vi "Analog Output Control Panel (No Objects).vi"(8 "error in (no error)":errorcluster) -> (0 "error out":errorcluster)   [LabVIEW 2009]
doc: "(Dynamic) A user-level application that simulates the physical front panel of the Instrument. Provide the user with buttons to manually control features of the instrument, and provide indicators of its current state."
uses:
  <vilib>/DAQmx/create/channels.llb/DAQmx Create Channel (AO-Voltage-Basic).vi
  <vilib>/DAQmx/write.llb/DAQmx Write (Analog DBL 1Chan 1Samp).vi
  Program Files/National Instruments/LabVIEW 2009/resource/objmgr/daqmx.rc
panel:
  in  "Copy actual to set":bool
  in  "Populate fields with member data":bool
  out "Ch1 voltage":dbl[unit]
  out "Ch1 lower limit":dbl[unit]
  out "Ch1 upper limit":dbl[unit]
  out "Ch0 voltage":dbl[unit]
  out "Ch0 lower limit":dbl[unit]
  out "Ch0 upper limit":dbl[unit]
  in  "Set Ch1 Voltage":bool
  in  "Set Ch0 Voltage":bool
  in  "Ch1 voltage set":dbl[unit]
  in  "Ch1 lower limit set":dbl[unit] min=-10.0 max=10.0
  in  "Ch1 upper limit set":dbl[unit] min=-10.0 max=10.0
  in  "Ch0 voltage set":dbl[unit]
  in  "Ch0 lower limit set":dbl[unit] min=-10.0 max=10.0
  in  "Ch0 upper limit set":dbl[unit] min=-10.0 max=10.0
  in  "Set Parameters":bool
  in  "Read to Control":bool
  in  "Read Parameters":bool
  in  "stop":bool
  # "We cannot read in the currently set voltage values !"
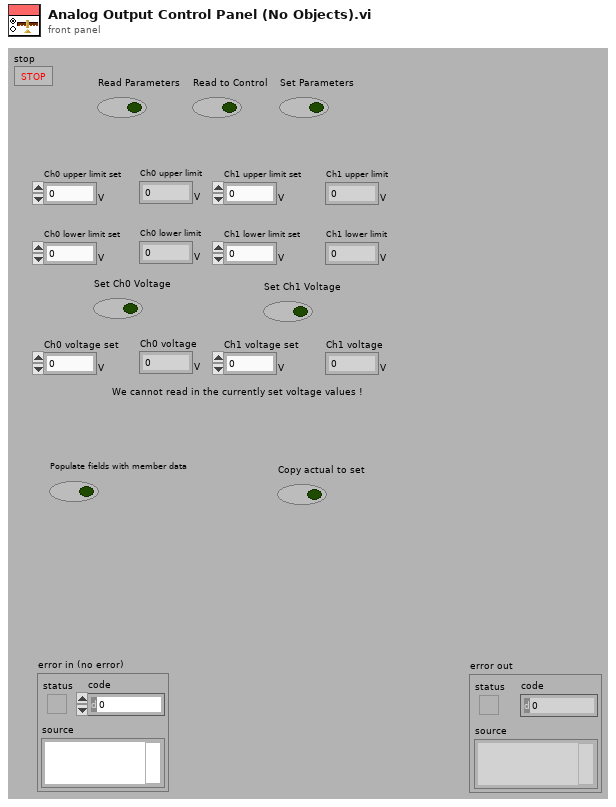
[diagram p1: front panel]
types:
  T1 = cluster{"Ch0":cluster{"Voltage":dbl[unit], "Max value":dbl[unit], "Min value":dbl[unit], "Ch 0 task":refnum<k21>}, "Ch1":cluster{"Voltage":dbl[unit], "Max value":dbl[unit], "Min value":dbl[unit], "Ch 1 task":refnum<k21>}}
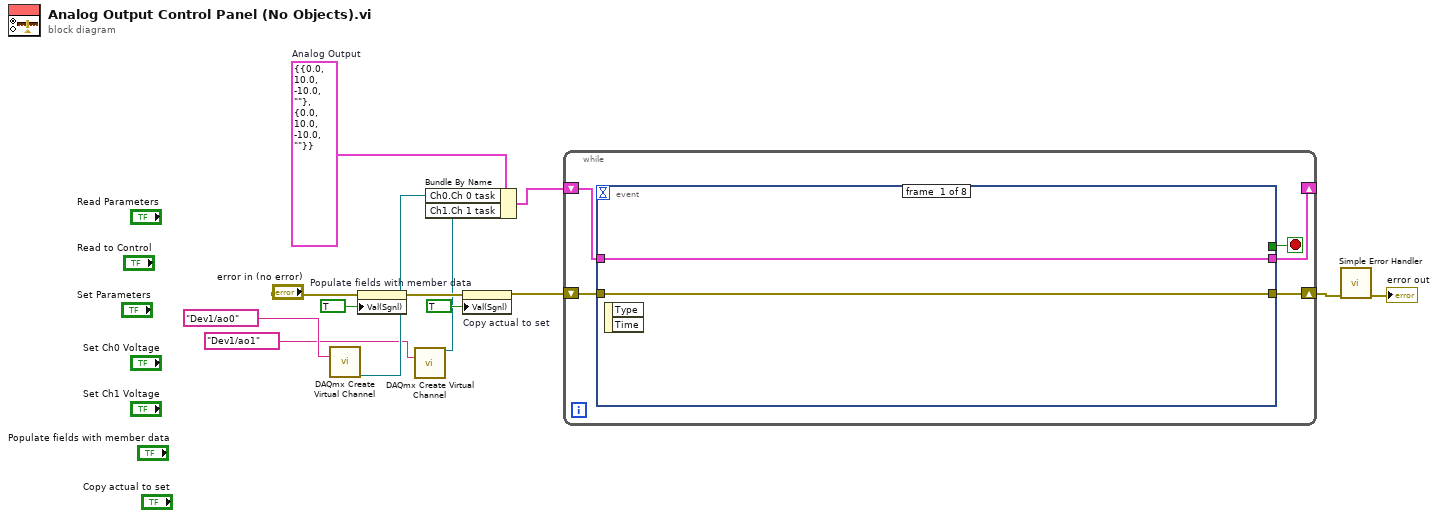
[diagram p0: block diagram]
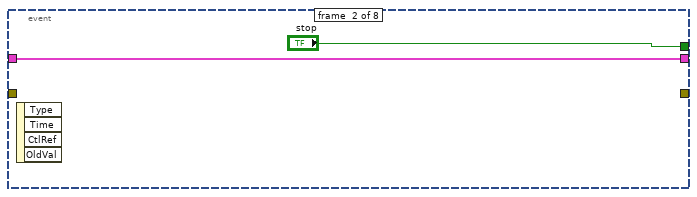
[diagram p2: hidden frame]
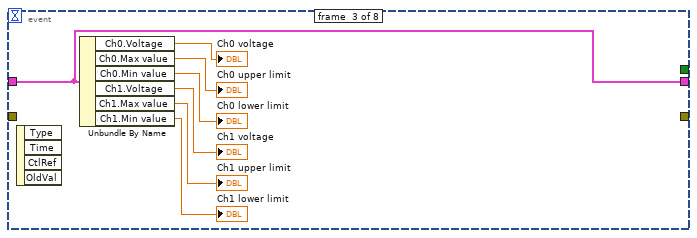
[diagram p3: hidden frame]
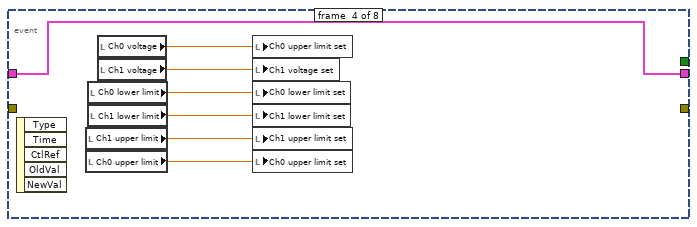
[diagram p4: hidden frame]
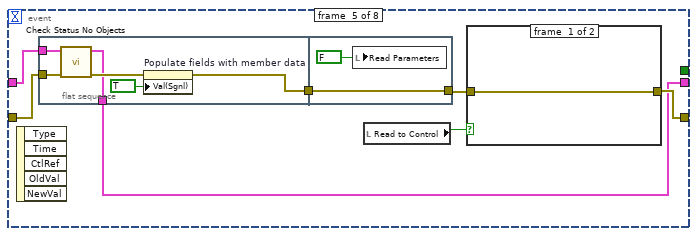
[diagram p5: hidden frame]
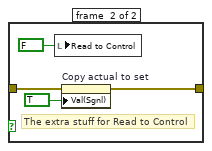
[diagram p6: hidden frame]
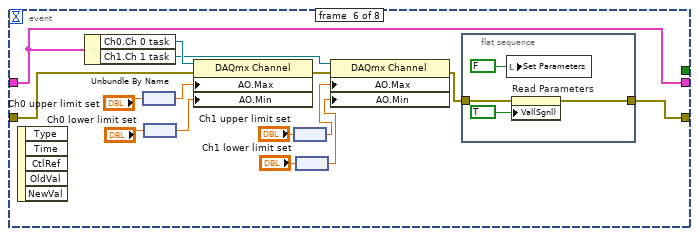
[diagram p7: hidden frame]
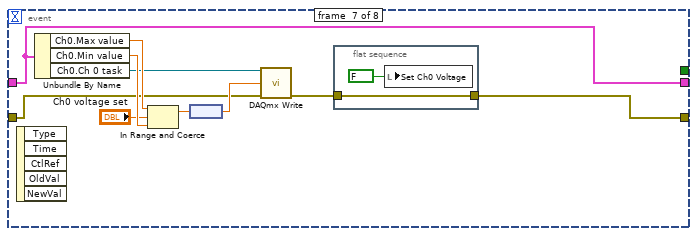
[diagram p8: hidden frame]
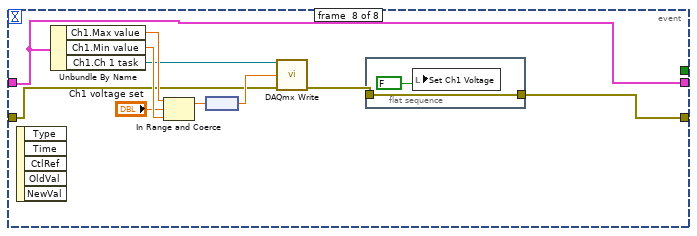
[diagram p9: hidden frame]
diagram:
  w6 = T1 {"Ch0"={"Voltage"=0.0, "Max value"=10.0, "Min value"=-10.0, "Ch 0 task"=""}, "Ch1"={"Voltage"=0.0, "Max value"=10.0, "Min value"=-10.0, "Ch 1 task"=""}}  # Analog Output
  n1 = call-poly <vilib>:"DAQmx Create Virtual Channel.vi"("physical channels"=tag "Dev1/ao0") -> ("task out"=w4:refnum<k21>)  [unwired: 13 in, 1 out]
  n2 = property on="Populate fields with member data" class="Bool (strict)"(error in="error in (no error)", "Val(Sgnl)"=TRUE ("Value (Signaling)")) -> (error out=w11:errorcluster)  [unwired: 1 in, 1 out]
  n3 = call-poly <vilib>:"DAQmx Create Virtual Channel.vi"("physical channels"=tag "Dev1/ao1") -> ("task out"=w3:refnum<k21>)  [unwired: 13 in, 1 out]
  n4 = Bundle By Name(cluster=w6, "Ch0.Ch 0 task"=w4, "Ch1.Ch 1 task"=w3) -> (w5:T1)
  n5 = property on="Copy actual to set" class="Bool (strict)"(error in=w11, "Val(Sgnl)"=TRUE ("Value (Signaling)")) -> (error out=w10:errorcluster)  [unwired: 1 in, 1 out]
  n6 = while {
    shift-right: [w14] -> _
    shift-left: w5 -> [w17]
    shift-right: [w16] -> w9
    shift-left: w10 -> [w18]
    stop <- w15 stop-if-true
    n7 = event shown="[4] \"Read Parameters\", \"Read to Control\": Value Change" {
      selector: _ -> [_ _ _ _ _ _ _ _]
      dyn-events: _ -> [_ _ _ _ _ _ _ _]
      timeout: _ -> [_ _ _ _ _ _ _ _]
      tunnel: [w20 _ _ _ w38 w57 w76 w88] -> w16
      tunnel: w18 -> [w20 _ _ _ w42 w71 w80 w92]
      tunnel: w17 -> [w19 w22 w23 w30 w43 w58 w77 w89]
      tunnel: [w19 w22 w23 w30 w37 w58 w77 w89] -> w14
      tunnel: [_ "stop" _ _ _ _ _ _] -> w15
      event #0 {
        n8 = event-data() -> ()  [unwired: 1 in, 2 out]
      }
      event #1 {
        n9 = event-data() -> ()  [unwired: 1 in, 4 out]
      }
      event #2 {
        n10 = event-data() -> ()  [unwired: 1 in, 4 out]
        n11 = Unbundle By Name(w23) -> ("Ch0.Voltage"=→"Ch0 voltage":dbl[unit], "Ch0.Max value"=→"Ch0 upper limit":dbl[unit], "Ch0.Min value"=→"Ch0 lower limit":dbl[unit], "Ch1.Voltage"=→"Ch1 voltage":dbl[unit], "Ch1.Max value"=→"Ch1 upper limit":dbl[unit], "Ch1.Min value"=→"Ch1 lower limit":dbl[unit])
      }
      event #3 {
        n12 = event-data() -> ()  [unwired: 1 in, 5 out]
        n13 = local read "Ch1 upper limit"() -> (w32:dbl[unit])
        n14 = local read "Ch0 upper limit"() -> (w35:dbl[unit])
        n15 = local read "Ch0 lower limit"() -> (w36:dbl[unit])
        n16 = local read "Ch1 lower limit"() -> (w33:dbl[unit])
        n17 = local read "Ch0 voltage"() -> (w34:dbl[unit])
        n18 = local read "Ch1 voltage"() -> (w31:dbl[unit])
        n19 = local write "Ch0 upper limit set"(w34) -> ()
        n20 = local write "Ch1 voltage set"(w31) -> ()
        n21 = local write "Ch0 lower limit set"(w36) -> ()
        n22 = local write "Ch1 lower limit set"(w33) -> ()
        n23 = local write "Ch1 upper limit set"(w32) -> ()
        n24 = local write "Ch0 upper limit set"(w35) -> ()
      }
      event #4 {
        n25 = event-data() -> ()  [unwired: 1 in, 5 out]
        n26 = flat-sequence {
          tunnel: w43 -> [w50]
          tunnel: w42 -> [w51]
          tunnel: [w53] -> w41
          tunnel: [w49] -> w37
          tunnel: [w55] -> w39
          tunnel: w41 -> [w55]
          frame #0 {
            n27 = call "Check Status No Objects.vi"("error in (no error)"=w51, "Analog Output in"=w50) -> ("error out"=w52:errorcluster, "Analog Output out"=w49:T1)  [unwired: 6 in, 2 out]
            n28 = property on="Populate fields with member data" class="Bool (strict)"(error in=w52, "Val(Sgnl)"=TRUE ("Value (Signaling)")) -> (error out=w53:errorcluster)  [unwired: 1 in, 1 out]
          }
          frame #1 {
            n29 = local write "Read Parameters"(FALSE ("Read Parameters")) -> ()
          }
        }
        n30 = local read "Read to Control"() -> (w40:bool)
        n31 = case shown="True" w40 {
          tunnel: w39 -> [w44 w47]
          tunnel: [w44 w46] -> w38
          frame #0 {
          }
          frame #1 {
            # "The extra stuff for Read to Control"
            n32 = local write "Read to Control"(FALSE ("Read to Control")) -> ()
            n33 = property on="Copy actual to set" class="Bool (strict)"(error in=w47, "Val(Sgnl)"=TRUE ("Value (Signaling)")) -> (error out=w46:errorcluster)  [unwired: 1 in, 1 out]
          }
        }
      }
      event #5 {
        n34 = event-data() -> ()  [unwired: 1 in, 5 out]
        n35 = Unbundle By Name(w58) -> ("Ch0.Ch 0 task"=w62:refnum<k21>, "Ch1.Ch 1 task"=w61:refnum<k21>)
        n36 = node("Ch0 upper limit set") -> (w69:dbl)
        n37 = node("Ch0 lower limit set") -> (w65:dbl)
        n38 = property class="DAQmx Channel"(reference=w62, error in=w71, "AO.Max"=w69, "AO.Min"=w65) -> (error out=w60:errorcluster)  [unwired: 1 out]
        n39 = node("Ch1 upper limit set") -> (w64:dbl)
        n40 = node("Ch1 lower limit set") -> (w63:dbl)
        n41 = property class="DAQmx Channel"(reference=w61, error in=w60, "AO.Max"=w64, "AO.Min"=w63) -> (error out=w59:errorcluster)  [unwired: 1 out]
        n42 = flat-sequence {
          tunnel: w59 -> [w74]
          tunnel: [w73] -> w57
          frame #0 {
            n43 = local write "Set Parameters"(FALSE ("Set Parameters")) -> ()
            n44 = property on="Read Parameters" class="Bool (strict)"(error in=w74, "Val(Sgnl)"=TRUE ("Value (Signaling)")) -> (error out=w73:errorcluster)  [unwired: 1 in, 1 out]
          }
        }
      }
      event #6 {
        n45 = event-data() -> ()  [unwired: 1 in, 5 out]
        n46 = Unbundle By Name(w77) -> ("Ch0.Max value"=w84:dbl[unit], "Ch0.Min value"=w83:dbl[unit], "Ch0.Ch 0 task"=w79:refnum<k21>)
        n47 = In Range and Coerce(upper limit=w84, x="Ch0 voltage set", lower limit=w83) -> (coerced(x)=w81:dbl[unit])  [unwired: 1 out]
        n48 = node(w81) -> (w85:dbl)
        n49 = call-poly <vilib>:"DAQmx Write.vi"("task/channels in"=w79, "data"=w85, "error in"=w80) -> ("error out"=w78:errorcluster)  [unwired: 10 in, 2 out]
        n50 = flat-sequence {
          tunnel: [w86] -> w76
          tunnel: w78 -> [w86]
          frame #0 {
            n51 = local write "Set Ch0 Voltage"(FALSE ("Set Ch0 Voltage")) -> ()
          }
        }
      }
      event #7 {
        n52 = event-data() -> ()  [unwired: 1 in, 5 out]
        n53 = Unbundle By Name(w89) -> ("Ch1.Max value"=w96:dbl[unit], "Ch1.Min value"=w95:dbl[unit], "Ch1.Ch 1 task"=w91:refnum<k21>)
        n54 = In Range and Coerce(upper limit=w96, x="Ch1 voltage set", lower limit=w95) -> (coerced(x)=w94:dbl[unit])  [unwired: 1 out]
        n55 = node(w94) -> (w97:dbl)
        n56 = call-poly <vilib>:"DAQmx Write.vi"("task/channels in"=w91, "data"=w97, "error in"=w92) -> ("error out"=w90:errorcluster)  [unwired: 10 in, 2 out]
        n57 = flat-sequence {
          tunnel: [w98] -> w88
          tunnel: w90 -> [w98]
          frame #0 {
            n58 = local write "Set Ch1 Voltage"(FALSE ("Set Ch1 Voltage")) -> ()
          }
        }
      }
    }
  }
  n59 = call <vilib>:"Simple Error Handler.vi"("error in (no error)"=w9) -> ("error out"=→"error out":errorcluster)  [unwired: 1 in, 7 out]
